vi "Set Item Label.vi"(8 "error in (no error)":errorcluster, 10 "Name":string, 11 "Variant in":variant) -> (0 "error out":errorcluster, 3 "Variant out":variant)   [LabVIEW 2020, in "Variant Data Manipulation.lvlib"]
uses:
  Variant Data Manipulation.lvlib
  <vilib>/Utility/Data Type/NI_Data Type.lvlib
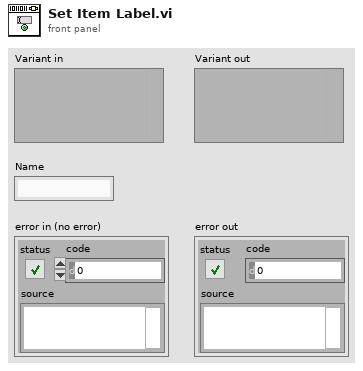
[diagram p1: front panel]
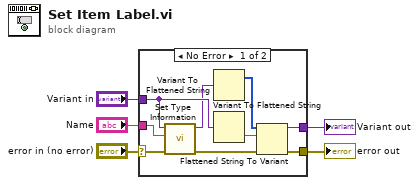
[diagram p0: block diagram]
diagram:
  n1 = case shown="No Error" "error in (no error)" {
    selector: "error in (no error)" -> [w8 w15]
    tunnel: "Variant in" -> [w14 w16]
    tunnel: [w10 w16] -> w2
    tunnel: "Name" -> [w9 _]
    tunnel: [w6 w15] -> w5
    frame No Error {
      n2 = call <vilib>:"Set Type Information.vi"("error in (no error)"=w8, "Name"=w9, "Variant in"=w14) -> ("error out"=w7:errorcluster, "Variant out"=w13:variant)  [unwired: 7 in]
      n3 = Variant To Flattened String(Variant=w13) -> (1:w12:i16[])  [unwired: 1 out]
      n4 = Variant To Flattened String(Variant=w14) -> (data string=w11:string)  [unwired: 1 out]
      n5 = Flattened String To Variant(4:w7, 6:w11, 7:w12) -> (0:w6:errorcluster, 3:w10:variant)
    }
    frame Error {
    }
  }
  "error out" <- w5
  "Variant out" <- w2
